vi "getCalibratedValueFromChannel.vi"(8 "error in (no error)":errorcluster, 9 "value":string, 10 "channel_name":string, 11 "ChannelArray in":refnum<class "ChannelArray.lvclass">) -> (0 "error out":errorcluster, 2 "calibratedValue":dbl, 3 "ChannelArray out":refnum<class "ChannelArray.lvclass">)   [LabVIEW 2009, in "Tools.lvlib" / "DatabaseHelpers.lvlib" / "ChannelArray.lvclass"]
uses:
  ChannelArray.lvclass
  Channel/Channel.lvclass
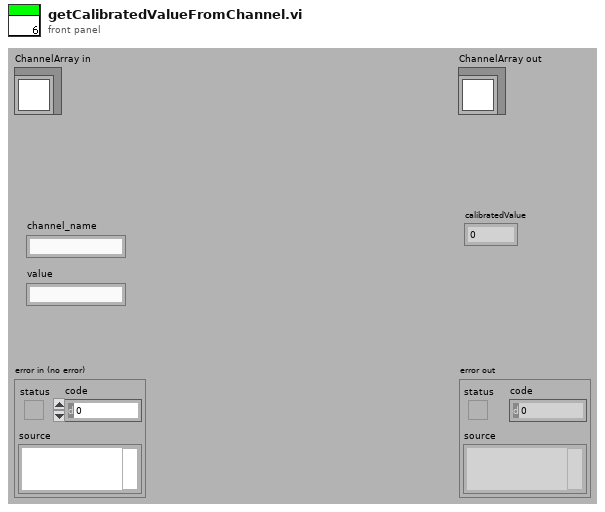
[diagram p1: front panel]
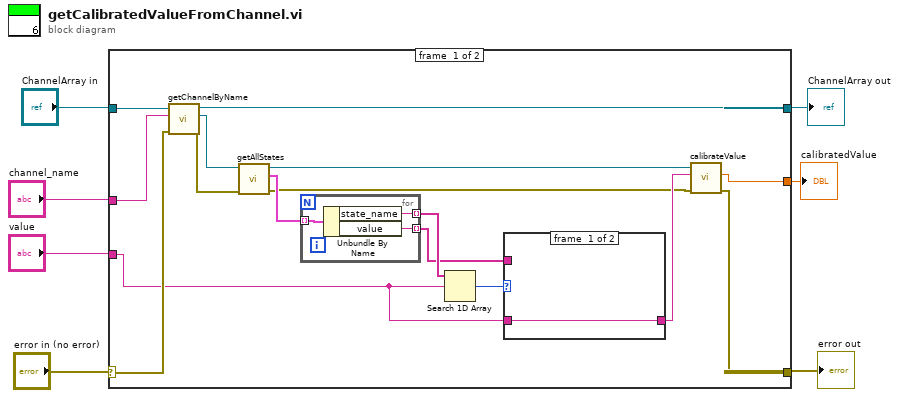
[diagram p0: block diagram]
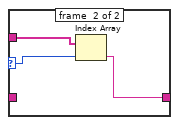
[diagram p2: hidden frame]
diagram:
  n1 = case shown="No Error" "error in (no error)" {
    selector: "error in (no error)" -> [w21 w32]
    tunnel: [w10 w32] -> w6
    tunnel: [w9 w31] -> w4
    tunnel: "ChannelArray in" -> [w23 w31]
    tunnel: "channel_name" -> [w22 _]
    tunnel: "value" -> [w15 _]
    tunnel: [w8 _] -> w1
    frame #0 {
      n2 = call-dynamic "getChannelByName.vi"("error in (no error)"=w21, "channel_name"=w22, "ChannelArray in"=w23) -> ("error out"=w11:errorcluster, "Channel"=w20:refnum<class "Channel.lvclass">, "ChannelArray out"=w9:refnum<class "ChannelArray.lvclass">)  [unwired: 5 in, 1 out]
      n3 = call "getAllStates.vi"("error in (no error)"=w11, "Channel.lvclass in"=w20) -> ("error out"=w12:errorcluster, "states"=w19:cluster{"state_name":string, "value":string}[], "Channel.lvclass out"=w14:refnum<class "Channel.lvclass">)  [unwired: 7 in]
      n4 = for {
        tunnel: w19 -> [w30] mode=indexing
        tunnel: [w29] -> w18 mode=indexing
        tunnel: [w28] -> w16 mode=indexing
        n5 = Unbundle By Name(w30) -> ("state_name"=w29:string, "value"=w28:string)
      }
      n6 = Search 1D Array(1D array=w18, element=w15) -> (index of element=w17:i32)  [unwired: 1 in]
      n7 = case shown="Default" w17 {
        selector: w17 -> [_ w26]
        tunnel: w16 -> [_ w27]
        tunnel: w15 -> [w24 _]
        tunnel: [w24 w25] -> w13
        frame #0 {
        }
        frame #1 {
          n8 = Index Array(array=w27, index=w26) -> (element=w25:string)
        }
      }
      n9 = call-dynamic "calibrateValue.vi"("error in (no error)"=w12, "value"=w13, "Channel in"=w14) -> ("error out"=w10:errorcluster, "calibratedValue"=w8:dbl)  [unwired: 6 in, 1 out]
    }
    frame #1 {
    }
  }
  "error out" <- w6
  "ChannelArray out" <- w4
  "calibratedValue" <- w1
